vi "G4BaseTemplate_Singleton_5x6x5_Init.vi"(0 "reference in":refnum<class "G4BaseTemplate_Singleton_5x6x5.lvclass"> caption="This control should only be used when\na sub class is inheriting this class", 11 "Error In":errorcluster) -> (4 "reference out":refnum<class "G4BaseTemplate_Singleton_5x6x5.lvclass"> caption="This indicator should only be used when\na sub class is inheriting this class", 15 "Error Out":errorcluster)   [LabVIEW 2020, in "G4BaseTemplate_Singleton_5x6x5.lvclass"]
uses:
  <resource>/Framework/Providers/Open_GDS/ClassProviders/Provider_EndevoGOOP400/Templates/G4BaseTemplate_Singleton_5x6x5/G4BaseTemplate_Singleton_5x6x5.lvclass
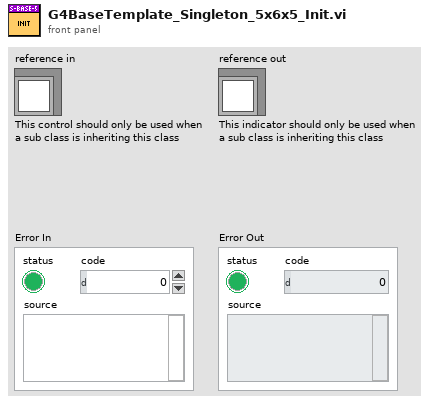
[diagram p1: front panel]
types:
  T1 = typedef "G4BaseTemplate_Singleton_5x6x5.lvclass/ObjectAttributes.ctl" = cluster{"Attribute1":dbl}
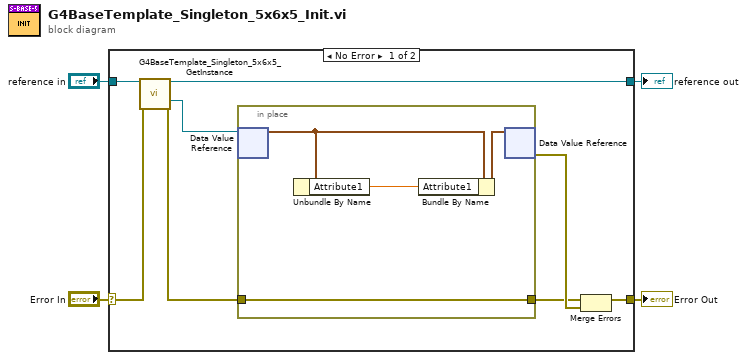
[diagram p0: block diagram]
diagram:
  n1 = case shown="No Error" "Error In" {
    selector: "Error In" -> [w10 w18]
    tunnel: [w11 w18] -> w3
    tunnel: "reference in" -> [w9 w17]
    tunnel: [w7 w17] -> w1
    frame No Error {
      n2 = call <resource>:"G4BaseTemplate_Singleton_5x6x5_GetInstance.vi"("reference in"=w9, "Error In"=w10) -> ("reference out"=w7:refnum<class "G4BaseTemplate_Singleton_5x6x5.lvclass">, "DVRRefOut"=w8:refnum<data-value>, "Error Out"=w6:errorcluster)  [unwired: 9 in, 2 out]
      n3 = in-place {
        in-place-border: w6 -> [w13]
        in-place-border: [w13] -> w5
        n4 = in-place-dvr #1(w8) -> (w15:T1)  [unwired: 1 out]
        n5 = Unbundle By Name(w15) -> ("Attribute1"=w14:dbl)
        n6 = Bundle By Name(cluster=w15, "Attribute1"=w14) -> (w16:T1)
        n7 = in-place-dvr #1(w16) -> (w12:errorcluster)  [unwired: 1 out]
      }
      n8 = Merge Errors(w5, w12) -> (w11:errorcluster)
    }
    frame Error {
    }
  }
  "Error Out" <- w3
  "reference out" <- w1
